vi "UI - Initiate Connection.vi"(8 "error in (no error)":errorcluster, 10 "Controller Address":string, 11 "Message Queue":refnum<queue>) -> (0 "error out":errorcluster, 1 "Connected?":bool)   [LabVIEW 2013]
uses:
  Message Queue/Message Cluster.ctl
  controls/Raw Values.ctl
  controls/FPGA State.ctl
  controls/Variable References.ctl
  Globals/Global - Configuration Options.vi
  Globals/Global - UI Stream and Variable Connections.vi
  Message Queue/Message Queue.lvlib
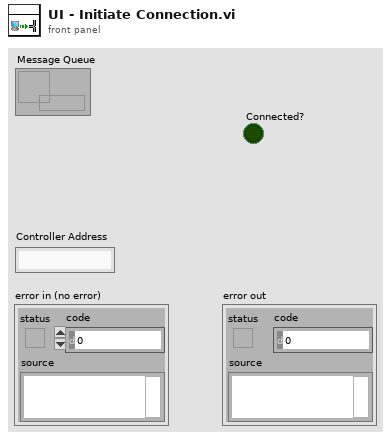
[diagram p1: front panel]
types:
  T1 = typedef "FPGA State.ctl" = enum16{"Safe State", "Manual", "Control (PID)"}
  T2 = typedef "Raw Values.ctl" = cluster{"Channel 0":fxp<+/-,20,5>, "Channel 1":fxp<+/-,20,5>, "Channel 2":fxp<+/-,20,5>, "Channel 3":fxp<+/-,20,5>}
  T3 = typedef "Message Queue.lvlib/Message Cluster.ctl" = cluster{"Message":string, "Message Data":variant}
  T4 = typedef "Variable References.ctl" = cluster{"CPU Usage":refnum<k21>, "Contiguous Memory":refnum<k21>, "Input Values":refnum<k21>, "Output Values":refnum<k21>, "FPGA Mode":refnum<k21>, "Actual Loop Period":refnum<k21>}
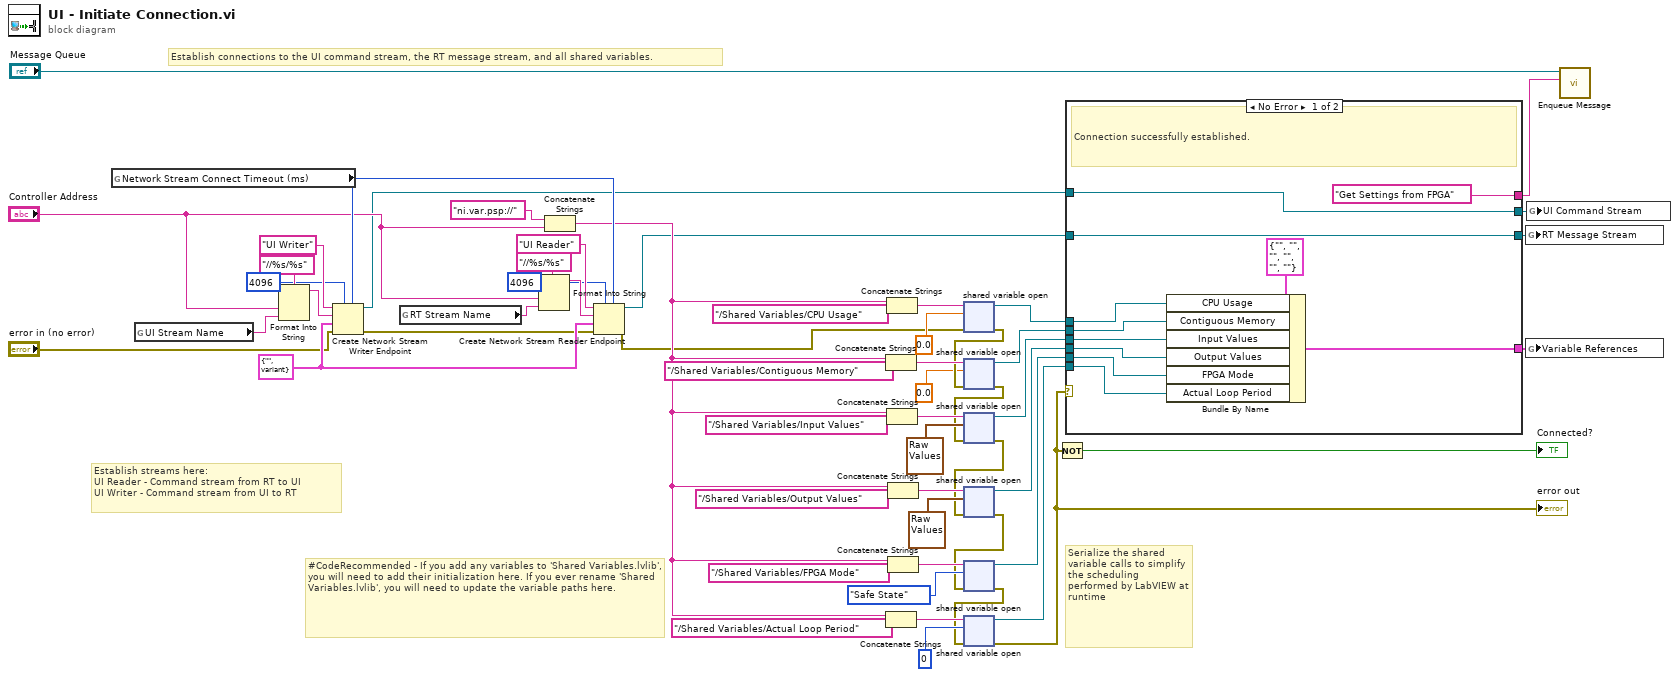
[diagram p0: block diagram]
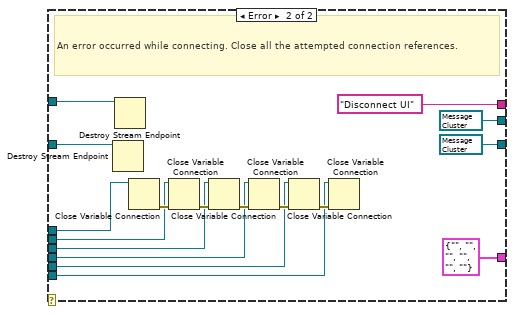
[diagram p2: hidden frame]
diagram:
  w47 = T3 {"Message"="", "Message Data"=variant} ("Message Cluster")
  # "Establish connections to the UI command stream, the RT message stream, and all shared variables."
  # "#CodeRecommended - If you add any variables to 'Shared Variables.lvlib', you will need to add their initialization here. If you ever rename 'Shared Variables.lvlib', you will need to update the variable paths here."
  # "Establish streams here:\nUI Reader - Command stream from RT to UI\nUI Writer - Command stream from UI to RT"
  # "Serialize the shared variable calls to simplify the scheduling performed by LabVIEW at runtime"
  n1 = global read "Global - Configuration Options.vi" "Network Stream Connect Timeout (ms)"() -> (w46:i32)
  n2 = global read "Global - Configuration Options.vi" "UI Stream Name"() -> (w54:string)
  n3 = Format Into String(format string="//%s/%s", "Controller Address", w54) -> (resulting string=w53:string)  [unwired: 2 in, 1 out]
  n4 = Create Network Stream Writer Endpoint(5:w46, 7:4096 ("writer buffer size"), 8:"error in (no error)", 9:w47, 10:w53, 11:"UI Writer" ("writer name")) -> (0:w5:errorcluster, 3:w13:refnum<k21>)  [unwired: 1 in]
  n5 = global read "Global - Configuration Options.vi" "RT Stream Name"() -> (w51:string)
  n6 = Format Into String(format string="//%s/%s", "Controller Address", w51) -> (resulting string=w50:string)  [unwired: 2 in, 1 out]
  n7 = Concatenate Strings("ni.var.psp://", "Controller Address") -> (w21:string)
  n8 = Create Network Stream Reader Endpoint(5:w46, 7:4096 ("reader buffer size"), 8:w5, 9:w47, 10:w50, 11:"UI Reader" ("reader name")) -> (0:w4:errorcluster, 3:w12:refnum<k21>)  [unwired: 1 in]
  n9 = Concatenate Strings(w21, "/Shared Variables/Contiguous Memory") -> (w39:string)
  n10 = Concatenate Strings(w21, "/Shared Variables/Actual Loop Period") -> (w31:string)
  n11 = Concatenate Strings(w21, "/Shared Variables/CPU Usage") -> (w42:string)
  n12 = Concatenate Strings(w21, "/Shared Variables/Input Values") -> (w37:string)
  n13 = Concatenate Strings(w21, "/Shared Variables/Output Values") -> (w35:string)
  n14 = Concatenate Strings(w21, "/Shared Variables/FPGA Mode") -> (w34:string)
  n15 = shared-variable-open(w42, w4, 0.0) -> (w19:refnum<k21>, w26:errorcluster)  [unwired: 1 in]
  n16 = shared-variable-open(w39, w26, 0.0) -> (w18:refnum<k21>, w25:errorcluster)  [unwired: 1 in]
  n17 = shared-variable-open(w37, w25, T2 {"Channel 0"=0.0, "Channel 1"=0.0, "Channel 2"=0.0, "Channel 3"=0.0}) -> (w17:refnum<k21>, w24:errorcluster)  [unwired: 1 in]
  n18 = shared-variable-open(w35, w24, T2 {"Channel 0"=0.0, "Channel 1"=0.0, "Channel 2"=0.0, "Channel 3"=0.0}) -> (w16:refnum<k21>, w23:errorcluster)  [unwired: 1 in]
  n19 = shared-variable-open(w34, w23, FPGA_State."Safe State" ("FPGA State")) -> (w15:refnum<k21>, w22:errorcluster)  [unwired: 1 in]
  n20 = shared-variable-open(w31, w22, u32 0) -> (w14:refnum<k21>, w20:errorcluster)  [unwired: 1 in]
  "error out" <- w20
  n21 = Not(x=w20) -> (.not. x?=→"Connected?":bool)
  n22 = case shown="No Error" w20 {
    tunnel: w19 -> [w66 w77]
    tunnel: w18 -> [w65 w72]
    tunnel: w17 -> [w64 w73]
    tunnel: w16 -> [w63 w74]
    tunnel: w15 -> [w62 w75]
    tunnel: w14 -> [w61 w76]
    tunnel: w13 -> [w57 w83]
    tunnel: w12 -> [w59 w84]
    tunnel: [w60 T4 {"CPU Usage"="", "Contiguous Memory"="", "Input Values"="", "Output Values"="", "FPGA Mode"="", "Actual Loop Period"=""} ("Variable References")] -> w11
    tunnel: [w59 refnum<k21> refnum] -> w10
    tunnel: [w57 refnum<k21> refnum] -> w9
    tunnel: ["Get Settings from FPGA" "Disconnect UI"] -> w7
    frame No Error {
      # "Connection successfully established."
      n23 = Bundle By Name(cluster=T4 {"CPU Usage"="", "Contiguous Memory"="", "Input Values"="", "Output Values"="", "FPGA Mode"="", "Actual Loop Period"=""} ("Variable References"), "CPU Usage"=w66, "Contiguous Memory"=w65, "Input Values"=w64, "Output Values"=w63, "FPGA Mode"=w62, "Actual Loop Period"=w61) -> (w60:T4)
    }
    frame Error {
      # "An error occurred while connecting. Close all the attempted connection references."
      n24 = Destroy Stream Endpoint(11:w84) -> ()  [unwired: 1 in, 1 out]
      n25 = Destroy Stream Endpoint(11:w83) -> ()  [unwired: 1 in, 1 out]
      n26 = Close Variable Connection(11:w77) -> (0:w78:errorcluster)  [unwired: 1 in]
      n27 = Close Variable Connection(8:w78, 11:w72) -> (0:w79:errorcluster)
      n28 = Close Variable Connection(8:w79, 11:w73) -> (0:w80:errorcluster)
      n29 = Close Variable Connection(8:w80, 11:w74) -> (0:w81:errorcluster)
      n30 = Close Variable Connection(8:w81, 11:w75) -> (0:w82:errorcluster)
      n31 = Close Variable Connection(8:w82, 11:w76) -> ()  [unwired: 1 out]
    }
  }
  n32 = global write "Global - UI Stream and Variable Connections.vi" "RT Message Stream"(w10) -> ()
  n33 = global write "Global - UI Stream and Variable Connections.vi" "Variable References"(w11) -> ()
  n34 = global write "Global - UI Stream and Variable Connections.vi" "UI Command Stream"(w9) -> ()
  n35 = call "Enqueue Message.vi"("Message"=w7, "Message Queue"="Message Queue") -> ()  [unwired: 8 in, 2 out]
